vi "open drive joystick.vi"   [LabVIEW 2019]
uses:
  <vilib>/Rock Robotics/WPI/Utilities/WPI_GetSetVariantRefNum.vi
  Robot Global Data.vi
types:
  T1 = typedef "WPI_JoystickDevRef.ctl" = cluster{"Device":T2}
  T2 = typedef "WPI_JoystickDeviceEnum.ctl" = enum16{"USB 0", "USB 1", "USB 2", "USB 3", "USB 4", "USB 5"}
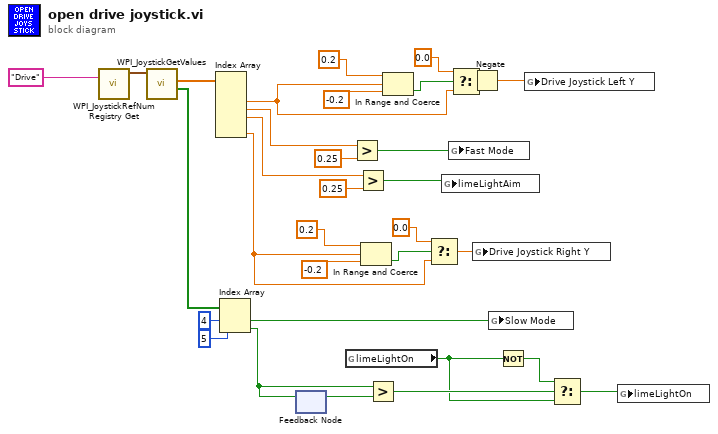
[diagram p0: block diagram]
diagram:
  n1 = call <vilib>:"WPI_JoystickRefNum Registry Get.vi"("refnum name"="Drive") -> ("JoystickDevRef"=w18:T1)  [unwired: 9 in, 1 out]
  n2 = call <vilib>:"WPI_JoystickGetValues.vi"("JoystickDevRef"=w18) -> ("Buttons"=w17:bool[], "Axes"=w31:dbl[])  [unwired: 6 in, 3 out]
  n3 = Index Array(array=w31) -> (element #2=w25:dbl, element #3=w15:dbl, element #4=w9:dbl, element #6=w19:dbl)  [unwired: 6 in, 2 out]
  n4 = Index Array(array=w17, index #1=4 ("index"), index #2=5 ("index")) -> (element #1=w12:bool, element #2=w4:bool)
  n5 = feedback-in #1(w4) -> ()
  n6 = feedback #1() -> (w3:bool)  [unwired: 1 in]
  n7 = global read "Robot Global Data.vi" "limeLightOn"() -> (w1:bool)
  n8 = Greater?(x=w15, y=0.25) -> (0:w13:bool)
  n9 = Greater?(x=w9, y=0.25) -> (0:w7:bool)
  n10 = In Range and Coerce(upper limit=0.2, x=w19, lower limit=-0.2) -> (In Range?=w20:bool)  [unwired: 1 out]
  n11 = Greater?(x=w4, y=w3) -> (0:w2:bool)
  n12 = In Range and Coerce(upper limit=0.2, x=w25, lower limit=-0.2) -> (In Range?=w26:bool)  [unwired: 1 out]
  n13 = Select(t=0.0, s=w20, f=w19) -> (s? t:f=w22:dbl)
  n14 = global write "Robot Global Data.vi" "limeLightAim"(w7) -> ()
  n15 = global write "Robot Global Data.vi" "Fast Mode"(w13) -> ()
  n16 = Select(t=0.0, s=w26, f=w25) -> (s? t:f=w28:dbl)
  n17 = Negate(x=w28) -> (-x=w11:dbl)
  n18 = global write "Robot Global Data.vi" "Drive Joystick Right Y"(w22) -> ()
  n19 = global write "Robot Global Data.vi" "Slow Mode"(w12) -> ()
  n20 = Not(x=w1) -> (.not. x?=w6:bool)
  n21 = global write "Robot Global Data.vi" "Drive Joystick Left Y"(w11) -> ()
  n22 = Select(t=w6, s=w2, f=w1) -> (s? t:f=w5:bool)
  n23 = global write "Robot Global Data.vi" "limeLightOn"(w5) -> ()
